vi "initialize debug mode.vi"(10 "User Event in":T1, 11 "editor node in":T2) -> (1 "engine":refnum<data-value>, 2 "User Event out":T1, 3 "editor node out":T2, 5 "Engine Configuration":refnum<class "engine configuration.lvclass">)   [LabVIEW 2014, in "configuration tests.lvlib" / "TEST EDITOR.lvclass"]
uses:
  TEST EDITOR.lvclass
  <vilib>/NI/Configuration Framework/Node/NodeRef.ctl
  <vilib>/NI/Configuration Framework/Node/NISE_CEF_Node.lvclass
  Configuration Editor/Classes/Engine Parent/Engine Parent Editor Node.lvclass
  <vilib>/NI/Configuration Framework/Node/UserEventRef.ctl
  <vilib>/NI/Configuration Framework/Controls/EventCluster.ctl
  <vilib>/NI/Module Execution Interface/Engine Configuration/engine configuration.lvclass
  Configuration Editor/Classes/Engine Parent/read engine configuration.vi
  Configuration Editor/Classes/Module editor node/module editor node.lvclass
  <vilib>/NI/Configuration Framework/NISE_CEF_TreeControl.lvlib
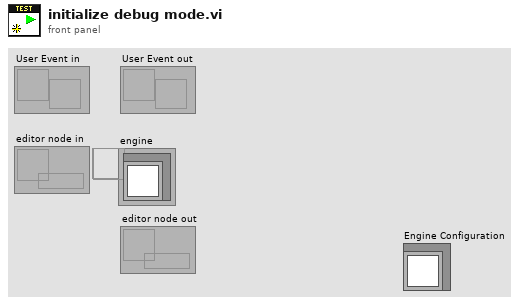
[diagram p1: front panel]
types:
  T1 = typedef "NISE_CEF_Node.lvclass/UserEventRef.ctl" = refnum<user-event>
  T2 = typedef "NISE_CEF_Node.lvclass/NodeRef.ctl" = refnum<data-value>
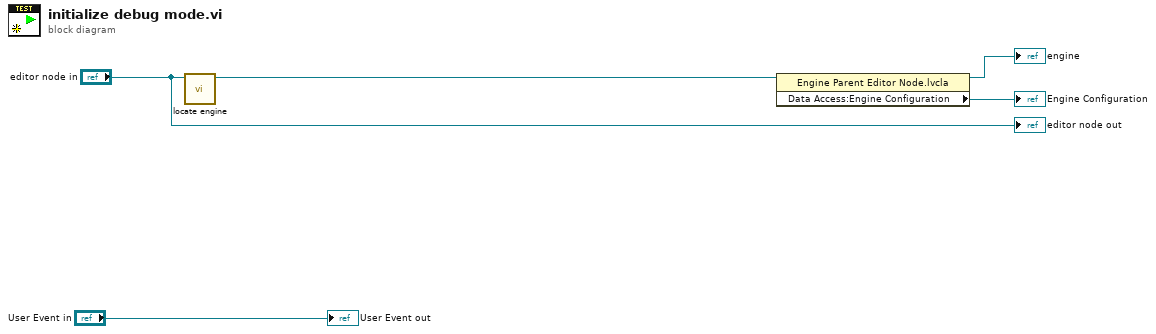
[diagram p0: block diagram]
diagram:
  n1 = call "locate engine.vi"("component"="editor node in") -> ("engine"=w1:refnum<data-value>)  [unwired: 9 in, 1 out]
  n2 = property class="Engine Parent Editor Node.lvcla"(reference=w1) -> (reference out=→"engine":refnum<data-value>, "Data Access:Engine Configuration"=→"Engine Configuration":refnum<class "engine configuration.lvclass">)  [unwired: 1 in, 1 out]
  "editor node out" <- "editor node in"
  "User Event out" <- "User Event in"
